vi "set_message.vi"(8 "error in (no error)":errorcluster, 9 "enqueue (back)":T1, 10 "message":string, 11 "timer in":refnum<class "rytimer.lvclass">) -> (0 "error out":errorcluster, 3 "timer out":refnum<class "rytimer.lvclass">)   [LabVIEW 2017, in "rytimer.lvclass"]
uses:
  rytimer.lvclass
  enqueue.ctl
  rytimer.lvclass/rytimer.ctl
  state.ctl
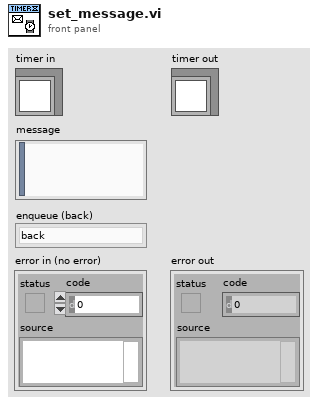
[diagram p1: front panel]
types:
  T1 = typedef "rytimer.lvclass/enqueue.ctl" = enum8{"back", "front", "back_if_absent", "front_if_absent"}
  T2 = typedef "rytimer.lvclass/state.ctl" = enum8{"stop", "start", "mode", "interval", "message"}
  T3 = cluster{"state":T2, "enqueue (back)":T1, "message":string}
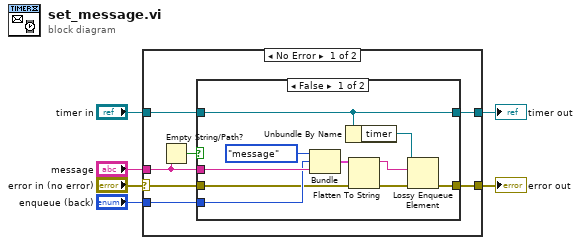
[diagram p0: block diagram]
diagram:
  n1 = case shown="No Error" "error in (no error)" {
    selector: "error in (no error)" -> [w12 w27]
    tunnel: "enqueue (back)" -> [w13 _]
    tunnel: "timer in" -> [w11 w26]
    tunnel: [w10 w27] -> w3
    tunnel: [w9 w26] -> w2
    tunnel: "message" -> [w8 _]
    frame No Error {
      n2 = Empty String/Path?(string/path=w8) -> (empty?=w7:bool)
      n3 = case shown="False" w7 {
        tunnel: w8 -> [w23 _]
        tunnel: w13 -> [w22 _]
        tunnel: w12 -> [w21 w24]
        tunnel: w11 -> [w14 w25]
        tunnel: [w20 w24] -> w10
        tunnel: [w14 w25] -> w9
        frame False {
          n4 = Bundle("state"=state."message", "enqueue (back)"=w22, "message"=w23) -> (w15:T3)  [unwired: 1 in]
          n5 = Unbundle By Name(w14) -> ("timer"=w19:refnum<queue>)
          n6 = Flatten To String(anything=w15, error in (no error)=w21) -> (data string=w16:string, error out=w17:errorcluster)  [unwired: 2 in, 1 out]
          n7 = Lossy Enqueue Element(queue=w19, element=w16, error in (no error)=w17) -> (error out=w20:errorcluster)  [unwired: 3 out]
        }
        frame True {
          # "Ignore invalid message"
        }
      }
    }
    frame Error {
    }
  }
  "error out" <- w3
  "timer out" <- w2
